vi "Save CSV (Async).vi"(5 "CSV File Ref":refnum<vi>, 7 "MONITOR TABLE Ref":refnum<vi>, 8 "error in (no error)":errorcluster, 11 "Measurement UI Queue":refnum<queue>) -> (0 "error out":errorcluster)   [LabVIEW 2025, in "I2C Bus Monitor UI.lvlib"]
uses:
  I2C Bus Monitor UI.lvlib
  Save CSV.vi
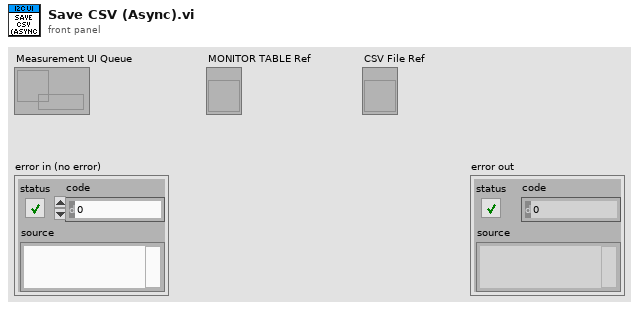
[diagram p1: front panel]
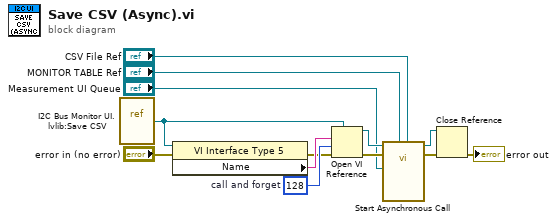
[diagram p0: block diagram]
diagram:
  w13 = 128  # call and forget
  n1 = vi-ref "I2C Bus Monitor UI.lvlib:Save CSV.vi"() -> (w6:refnum<vi>)
  n2 = property class="VI Interface Type 5"(reference=w6, error in="error in (no error)") -> (error out=w7:errorcluster, "Name"=w8:string)  [unwired: 1 out]
  n3 = Open VI Reference(type specifier VI Refnum (for type only)=w6, vi path=w8, options=w13, error in (no error)=w7) -> (vi reference=w12:refnum<vi>, error out=w11:errorcluster)  [unwired: 2 in]
  n4 = call-by-ref "Start Asynchronous Call"(reference=w12, error in=w11, "CSV FILE PATH Ref"="CSV File Ref", "MONITOR TABLE Ref"="MONITOR TABLE Ref", "Measurement UI Queue"="Measurement UI Queue") -> (reference out=w9:refnum<vi>, error out=w10:errorcluster)  [unwired: 8 in, 1 out]
  n5 = Close Reference(reference=w9, error in (no error)=w10) -> (error out=→"error out":errorcluster)
